vi "read_6dof_cal.vi"(8 "error in":errorcluster, 11 "Path":path) -> (0 "error out":errorcluster, 3 "6DOF Calibration":T1)   [LabVIEW 2024]
uses:
  6dof_calibration.ctl
panel:
  # "Read 6DOF calibration data from Matlab in text format, see ilemt/matlab/calibration/save_text_calibration.m"
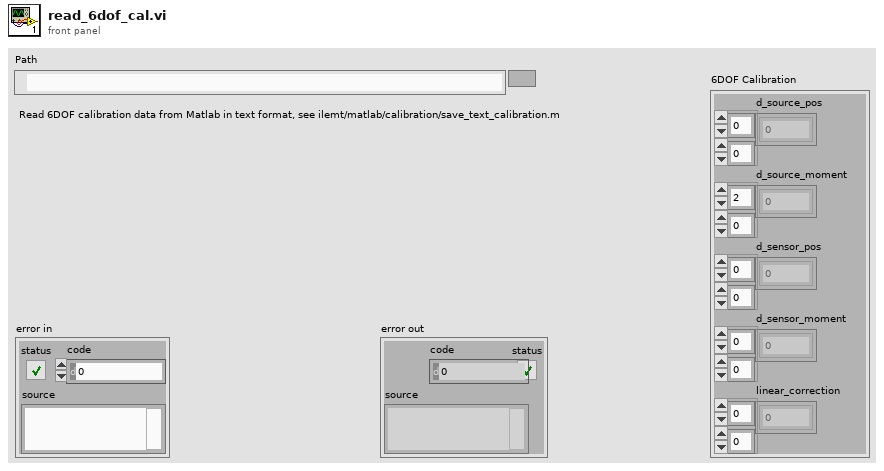
[diagram p1: front panel]
types:
  T1 = typedef "6dof_calibration.ctl" = cluster{"d_source_pos":dbl[][], "d_source_moment":dbl[][], "d_sensor_pos":dbl[][], "d_sensor_moment":dbl[][], "linear_correction":dbl[][]}
  T2 = cluster{"Result":dbl[][], "Result":dbl[][], "Result":dbl[][], "Result":dbl[][], "Result":dbl[][]}
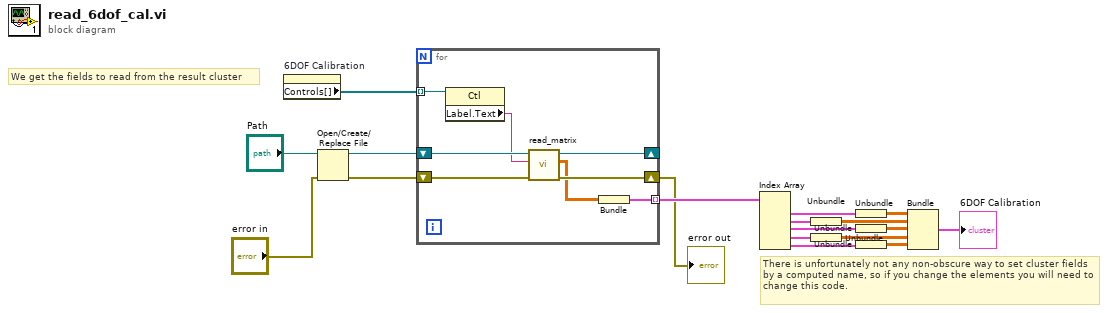
[diagram p0: block diagram]
diagram:
  # "We get the fields to read from the result cluster"
  # "There is unfortunately not any non-obscure way to set cluster fields by a computed name, so if you change the elements you will need to change this code."
  n1 = property on="6DOF Calibration" class="Clust (strict)"() -> ("Controls[]"=w14:refnum<vi>[])  [unwired: 2 in, 2 out]
  n2 = Open/Create/Replace File(file path (use dialog)="Path", error in="error in") -> (refnum out=w15:refnum<file>, error out=w16:errorcluster)  [unwired: 4 in, 1 out]
  n3 = for {
    tunnel: w14 -> [w24] mode=indexing
    shift-right: [w21] -> _
    shift-left: w15 -> [w25]
    shift-right: [w22] -> w1
    shift-left: w16 -> [w26]
    tunnel: [w19] -> w13 mode=indexing
    n4 = property class="Ctl"(reference=w24) -> ("Label.Text"=w23:string)  [unwired: 1 in, 2 out]
    n5 = call "read_matrix.vi"("error in"=w26, "Entry name"=w23, "file refnum"=w25) -> ("error out"=w22:errorcluster, "Result"=w20:dbl[][], "refnum out"=w21:refnum<file>)  [unwired: 4 in, 2 out]
    n6 = Bundle("Result"=w20) -> (w19:cluster{"Result":dbl[][]})  [unwired: 1 in]
  }
  "error out" <- w1
  n7 = Index Array(array=w13) -> (element #1=w12:cluster{"Result":dbl[][]}, element #2=w11:cluster{"Result":dbl[][]}, element #3=w9:cluster{"Result":dbl[][]}, element #4=w10:cluster{"Result":dbl[][]}, element #5=w8:cluster{"Result":dbl[][]})  [unwired: 5 in]
  n8 = Unbundle(w11) -> ("Result"=w6:dbl[][])
  n9 = Unbundle(w10) -> ("Result"=w4:dbl[][])
  n10 = Unbundle(w12) -> ("Result"=w7:dbl[][])
  n11 = Unbundle(w9) -> ("Result"=w5:dbl[][])
  n12 = Unbundle(w8) -> ("Result"=w3:dbl[][])
  n13 = Bundle("Result"=w7, "Result"=w6, "Result"=w5, "Result"=w4, "Result"=w3) -> (→"6DOF Calibration":T2)  [unwired: 1 in]
